vi "pad array.vi"(8 "X Step":dbl=0.00025 format="%#_13g", 9 "min value":dbl, 10 "max value":dbl, 11 "G 2":cluster{dbl[], dbl[]}(graph)) -> (3 "G 3":cluster{dbl[], dbl[]}(graph))   [LabVIEW 2016]
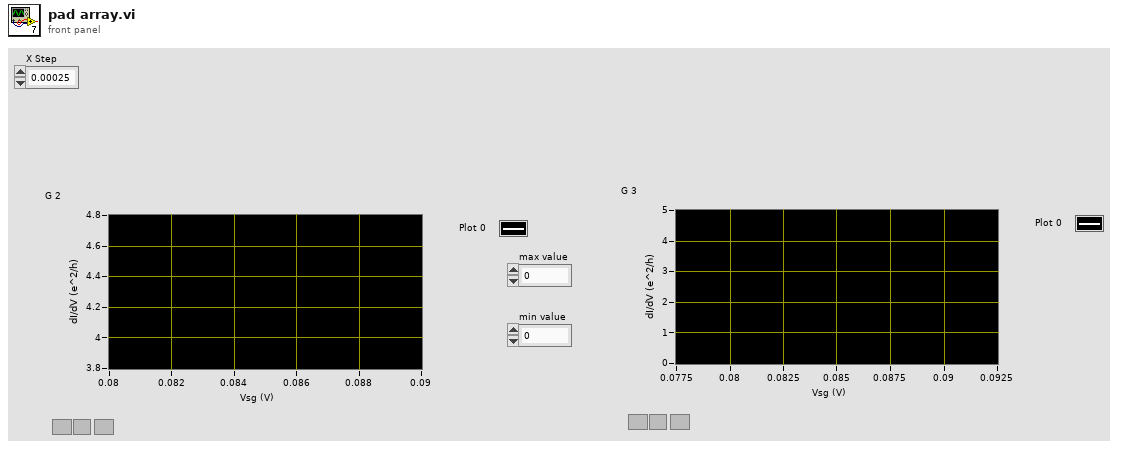
[diagram p1: front panel]
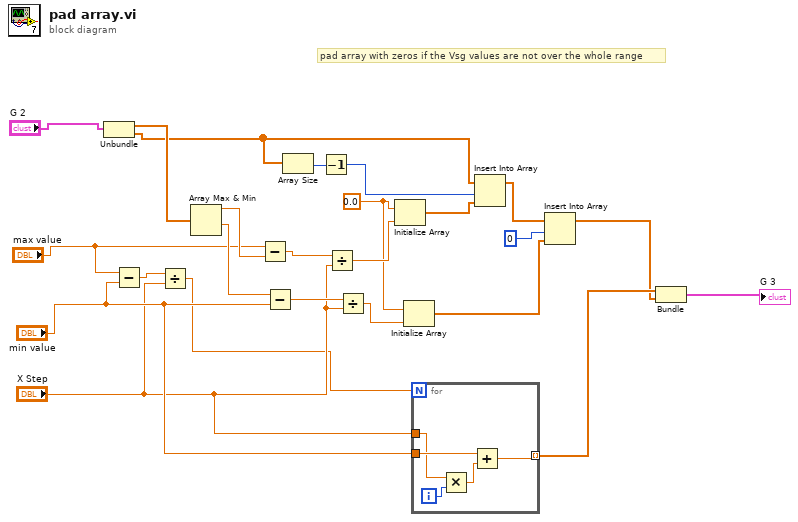
[diagram p0: block diagram]
diagram:
  w14 = 0.0
  # "pad array with zeros if the Vsg values are not over the whole range"
  n1 = Unbundle("G 2") -> (w15:dbl[], w10:dbl[])
  n2 = Subtract(x="max value", y="min value") -> (x-y=w7:dbl)
  n3 = Divide(x=w7, y="X Step") -> (x/y=w5:dbl)
  n4 = Array Max & Min(array=w15) -> (max value=w23:dbl, min value=w22:dbl)  [unwired: 2 out]
  n5 = Subtract(x="max value", y=w23) -> (x-y=w21:dbl)
  n6 = Subtract(x=w22, y="min value") -> (x-y=w20:dbl)
  n7 = Array Size(array=w10) -> (size(s)=w17:i32)
  n8 = Decrement(x=w17) -> (x-1=w16:i32)
  n9 = Divide(x=w21, y="X Step") -> (x/y=w19:dbl)
  n10 = Divide(x=w20, y="X Step") -> (x/y=w13:dbl)
  n11 = Initialize Array(w14, w19) -> (w18:dbl[])
  n12 = Initialize Array(w14, w13) -> (w12:dbl[])
  n13 = for {
    N: w5 -> [_]
    tunnel: "min value" -> [w29]
    tunnel: "X Step" -> [w27]
    tunnel: [w25] -> w4 mode=indexing
    i -> [w28]
    n14 = Multiply(x=w27, y=w28) -> (x*y=w26:dbl)
    n15 = Add(x=w29, y=w26) -> (x+y=w25:dbl)
  }
  n16 = Insert Into Array(array=w10, index=w16, new element=w18) -> (w3:dbl[])
  n17 = Insert Into Array(array=w3, index=0, new element=w12) -> (w2:dbl[])
  n18 = Bundle(w4, w2) -> (→"G 3":cluster{dbl[], dbl[]})  [unwired: 1 in]
